vi "API - Generate Tx Timestamp Channel.vi"(6 "New Header Config":bool[](array[boolean]), 7 "Previous Header Config":bool[](array[boolean]), 8 "error in (no error)":errorcluster, 11 "Packet Ref in":T1 format="%.0x") -> (0 "error out":errorcluster, 3 "Packet Ref out":T1 format="%.0x")   [LabVIEW 2016, in "UDP-Custom-Device System Explorer.lvlib"]
uses:
  UDP-Custom-Device System Explorer.lvlib
  <vilib>/NI Veristand/Custom Device API/Custom Device Item Ref.ctl
  <vilib>/NI Veristand/Custom Device API/Custom Device Channel.ctl
  <vilib>/NI Veristand/Custom Device API/Custom Device Channel Type.ctl
  Shared/Constants.vi
  <vilib>/NI VeriStand/Custom Device API/Custom Device API.lvlib
  Shared/UDP-Custom-Device Shared.lvlib
  <vilib>/NI VeriStand/Custom Device Tools/Custom Device Utility Library/Custom Device Utility Library.lvlib
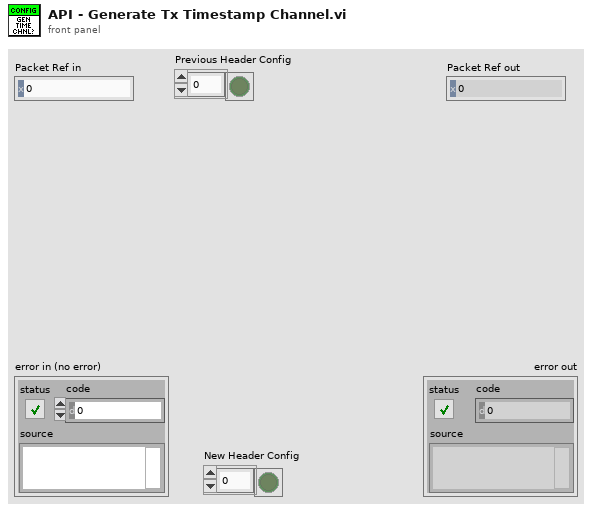
[diagram p1: front panel]
types:
  T1 = typedef "Custom Device API.lvlib/Custom Device Item Ref.ctl" = u64
  T2 = typedef "Custom Device API.lvlib/Custom Device Channel.ctl" = cluster{"Type":T3, "Units":string, "Default Value":dbl, "Faultable":bool, "Scalable":bool}
  T3 = typedef "Custom Device API.lvlib/Custom Device Channel Type.ctl" = enum16{"Input", "Output"}
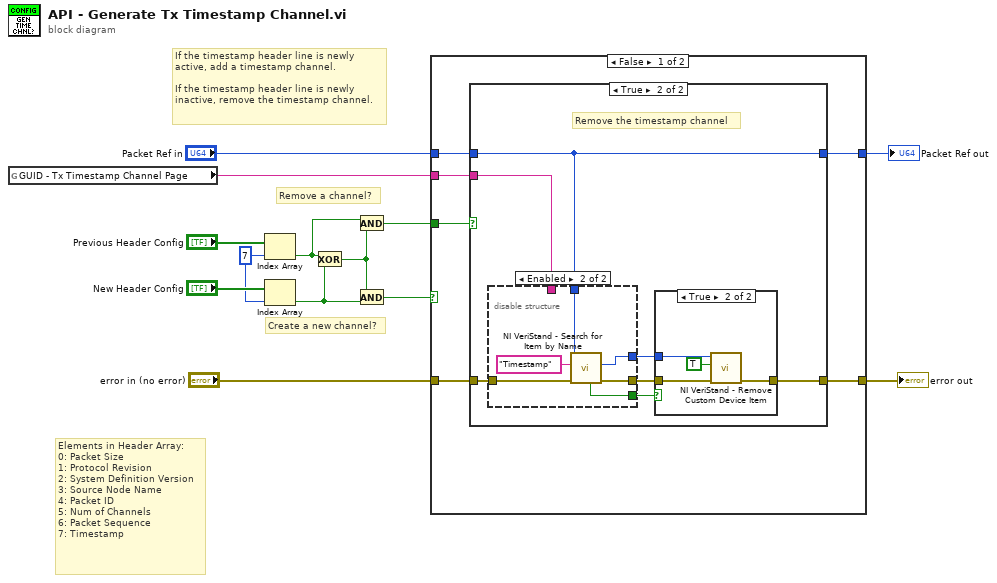
[diagram p0: block diagram]
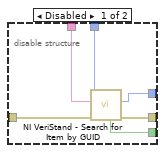
[diagram p3: hidden frame]
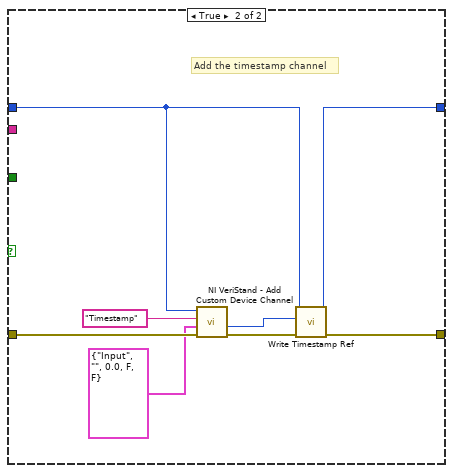
[diagram p5: hidden frame]
diagram:
  w11 = 7 ("index")
  # "If the timestamp header line is newly\nactive, add a timestamp channel.\n\nIf the timestamp header line is newly\ninactive, remove the timestamp channel."
  # "Remove a channel?"
  # "Create a new channel?"
  # "Elements in Header Array:\n0: Packet Size\n1: Protocol Revision\n2: System Definition Version\n3: Source Node Name\n4: Packet ID\n5: Num of Channels\n6: Packet Sequence\n7: Timestamp"
  n1 = global read "Constants.vi" "GUID - Tx Timestamp Channel Page"() -> (w1:string)
  n2 = Index Array(array="Previous Header Config", index=w11) -> (element=w7:bool)
  n3 = Index Array(array="New Header Config", index=w11) -> (element=w10:bool)
  n4 = Exclusive Or(1:w10, 2:w7) -> (0:w8:bool)
  n5 = And(x=w7, y=w8) -> (x .and. y?=w6:bool)
  n6 = And(x=w8, y=w10) -> (x .and. y?=w9:bool)
  n7 = case shown="False" w9 {
    tunnel: w6 -> [w19 _]
    tunnel: "Packet Ref in" -> [w18 w50]
    tunnel: [w15 w49] -> w4
    tunnel: [w17 w47] -> w3
    tunnel: "error in (no error)" -> [w16 w53]
    tunnel: w1 -> [w14 _]
    frame False {
      n8 = case shown="True" w19 {
        tunnel: w18 -> [w21 w27]
        tunnel: [w20 w28] -> w17
        tunnel: w16 -> [w20 w25]
        tunnel: [w21 w27] -> w15
        tunnel: w14 -> [_ w26]
        frame False {
        }
        frame True {
          # "Remove the timestamp channel"
          n9 = disable-structure shown="Enabled" {
            disable-tunnel: w27 -> [w34 w40]
            disable-tunnel: w26 -> [w33 _]
            disable-tunnel: w25 -> [w32 w37]
            disable-tunnel: [w31 w38] -> w24
            disable-tunnel: [w30 w39] -> w23
            disable-tunnel: [w29 w35] -> w22
            frame Disabled {
              n10 = call <vilib>:"NI VeriStand - Search for Item by GUID.vi"("error in"=w32, "Item GUID"=w33, "Section Ref in"=w34) -> ("error out"=w31:errorcluster, "Item Ref"=w30:T1, "Found"=w29:bool)  [unwired: 5 in, 1 out]
            }
            frame Enabled {
              n11 = call <vilib>:"NI VeriStand - Search for Item by Name.vi"("error in"=w37, "Item Name"="Timestamp", "Section Ref in"=w40) -> ("error out"=w38:errorcluster, "Item Ref"=w39:T1, "Found"=w35:bool)  [unwired: 5 in, 1 out]
            }
          }
          n12 = case shown="True" w22 {
            tunnel: [w41 w44] -> w28
            tunnel: w24 -> [w41 w43]
            tunnel: w23 -> [_ w42]
            frame False {
            }
            frame True {
              n13 = call <vilib>:"NI VeriStand - Remove Custom Device Item.vi"("error in (no error)"=w43, "Force Delete (F)"=TRUE, "Item Ref in"=w42) -> ("error out"=w44:errorcluster)  [unwired: 7 in, 1 out]
            }
          }
        }
      }
    }
    frame True {
      # "Add the timestamp channel"
      n14 = call <vilib>:"NI VeriStand - Add Custom Device Channel.vi"("error in (no error)"=w53, "Channel"=T2 {"Type"=enum."Input", "Units"="", "Default Value"=0.0, "Faultable"=FALSE, "Scalable"=FALSE}, "Channel Name"="Timestamp", "Parent Ref in"=w50) -> ("error out"=w48:errorcluster, "Channel Ref"=w46:T1)  [unwired: 4 in, 2 out]
      n15 = call "Write Timestamp Ref.vi"("error in (no error)"=w48, "Dependent Node Ref"=w46, "Node Ptr"=w50) -> ("error out"=w47:errorcluster, "Node Ptr out"=w49:T1)  [unwired: 7 in]
    }
  }
  "error out" <- w3
  "Packet Ref out" <- w4
